vi "1. Opening the Box.vi"() -> ()   [LabVIEW 2023]
uses:
  Box/Box.lvclass
  Flathead/Flathead.lvclass
  c:/dev/_r/4/eng/lv-core/lvpostprocessingd/lv_mc_x86_64/dist_i386/examples/Object-Oriented Programming/Basic Interfaces/Lever/Lever.lvclass
  Nailer/Nailer.lvclass
  Prybar/Prybar.lvclass
  c:/dev/_r/4/eng/lv-core/lvpostprocessingd/lv_mc_x86_64/dist_i386/examples/Object-Oriented Programming/Basic Interfaces/Prying Tool/Prying Tool.lvclass
  Bottle Opener/Bottle Opener.lvclass
  House Key/House Key.lvclass
  Prybar/Prybar.lvclass/Prybar.ctl
  Box/Box State.ctl
  Box/Box.lvclass/Box.ctl
  Prying Tool/Prying Tool.lvclass
panel:
  in  "format string":string="After %d attempts, the box is %s."
  out "Box":refnum<class "Box.lvclass">
  in  "force in Newtons":dbl=10.0
  # "Overview: This application demonstrates one of the uses of LabVIEW interfaces. It shows how an interface may be used to represent a common role in the system and then allow multiple classes to fulfill that role.\n\nDetail: This example starts with a box. The box is sealed but has a small crack in it where it can be wedged open with the right tool and enough force. The example explores how this can be modeled in software. \n\nAn interface can be thought of as a class without a private data control, but that small difference enables an interface to serve entirely different purposes in software architectures than classes. Specifically, interfaces enable a form of multiple inheritance. An interface declares a role that an object can play without defining how to perform that role. By inheriting from an interface, a class declares that its objects fulfill that role and the class becomes responsible for specifying how the behaviors are performed. When a class inherits from multiple interfaces, its objects can be passed into multiple software modules requiring different roles.\n \nInstructions:\n1. Select View>>LabVIEW Class Hierarchy to see the inheritance tree in this example. Notice that some items have multiple parents. A class may inherit from only one parent class but as many parent interfaces as needed for its role in the software. Inheriting from an interface allows that class to be wired to any terminal of that interface type.\n2. Open the block diagram and refer to the comments there.\n3. Run the VI after reading the comments. The runtime behavior will make more sense then."
  # "This is how much force you apply using the tools to try to open the box. Changing force will change which tools can successfully open the box."
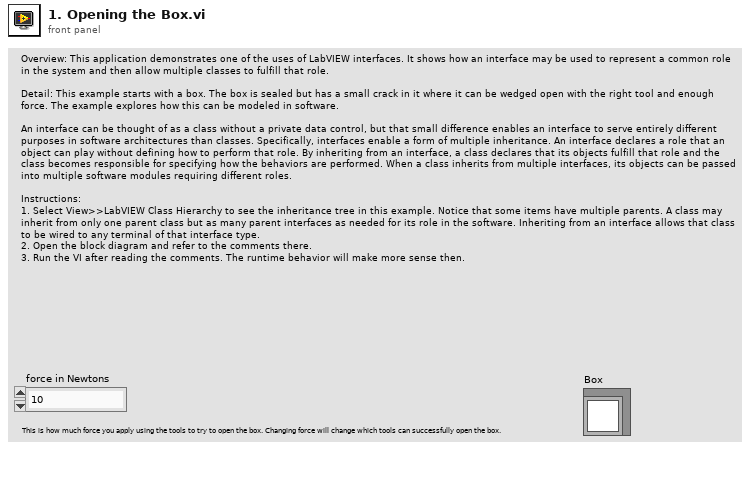
[diagram p1: front panel]
types:
  T1 = typedef "Box.lvclass/Box State.ctl" = enum16{"Closed", "Open"}
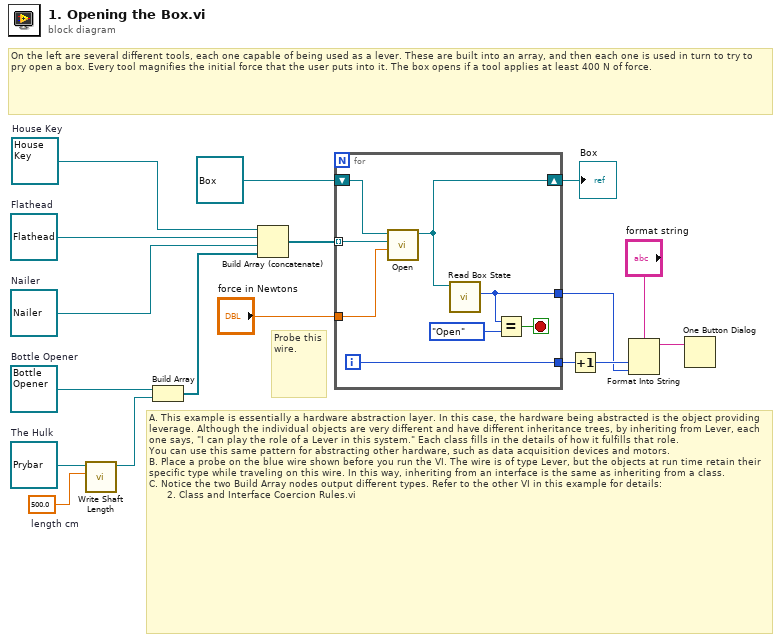
[diagram p0: block diagram]
diagram:
  w1 = refnum<class "House Key.lvclass"> refnum  # House Key
  w4 = refnum<class "Bottle Opener.lvclass"> refnum  # Bottle Opener
  w5 = refnum<class "Prybar.lvclass"> refnum  # The Hulk
  w15 = 500.0  # length cm
  w16 = refnum<class "Nailer.lvclass"> refnum  # Nailer
  w17 = refnum<class "Flathead.lvclass"> refnum  # Flathead
  # "Probe this wire."
  # "A. This example is essentially a hardware abstraction layer. In this case, the hardware being abstracted is the object providing leverage. Although the individual objects are very different and have different inheritance trees, by inheriting from Lever, each one says, \"I can play the role of a Lever in this system.\" Each class fills in the details of how it fulfills that role.\nYou can use this same pattern for abstracting other hardware, such as data acquisition devices and motors.\nB. Place a probe on the blue wire shown before you run the VI. The wire is of type Lever, but the objects at run time retain their specific type while traveling on this wire. In this way, inheriting from an interface is the same as inheriting from a class.\nC. Notice the two Build Array nodes output different types. Refer to the other VI in this example for details:\n      2. Class and Interface Coercion Rules.vi"
  # "On the left are several different tools, each one capable of being used as a lever. These are built into an array, and then each one is used in turn to try to pry open a box. Every tool magnifies the initial force that the user puts into it. The box opens if a tool applies at least 400 N of force."
  n1 = call "Write Shaft Length.vi"("length cm"=w15, "Prybar in"=w5) -> ("Prybar out"=w3:refnum<class "Prybar.lvclass">)  [unwired: 9 in]
  n2 = Build Array(w4, w3) -> (w2:refnum<class "Prying Tool.lvclass">[])
  n3 = Build Array (concatenate)(w1, w17, w16, w2) -> (w13:refnum<class "Lever.lvclass">[])
  n4 = for {
    tunnel: w13 -> [w24] mode=indexing
    shift-right: [w22] -> w11
    shift-left: refnum<class "Box.lvclass"> refnum ("Box.lvclass") -> [w25]
    tunnel: "force in Newtons" -> [w23]
    tunnel: [w19] -> w10
    tunnel: [w18] -> w7
    i -> [w19]
    stop <- w20 stop-if-true
    n5 = call "Open.vi"("force"=w23, "Lever"=w24, "Box in"=w25) -> ("Box out"=w22:refnum<class "Box.lvclass">)  [unwired: 8 in]
    n6 = call "Read Box State.vi"("Box in"=w22) -> ("box state"=w18:T1)  [unwired: 10 in]
    n7 = Equal?(x=w18, y=Box_State."Open") -> (x = y?=w20:bool)
  }
  "Box" <- w11
  n8 = Increment(x=w10) -> (x+1=w9:i32)
  n9 = Format Into String(format string="format string", w9, w7) -> (resulting string=w6:string)  [unwired: 2 in, 1 out]
  n10 = One Button Dialog(message=w6) -> ()  [unwired: 1 in, 1 out]
